vi "ReadText.vi"(8 "error in (no error)":errorcluster caption="错误输入（无错误）", 11 "zsActor输入":refnum<class "zsActor.lvclass">) -> (0 "error out":errorcluster caption="错误输出", 2 "Text":refnum<user-event>, 3 "zsActor输出":refnum<class "zsActor.lvclass">)   [LabVIEW 2014, in "Wrapper.lvlib" / "zsActor.lvclass"]
uses:
  zsActor.lvclass
  zsActor.lvclass/zsActor.ctl
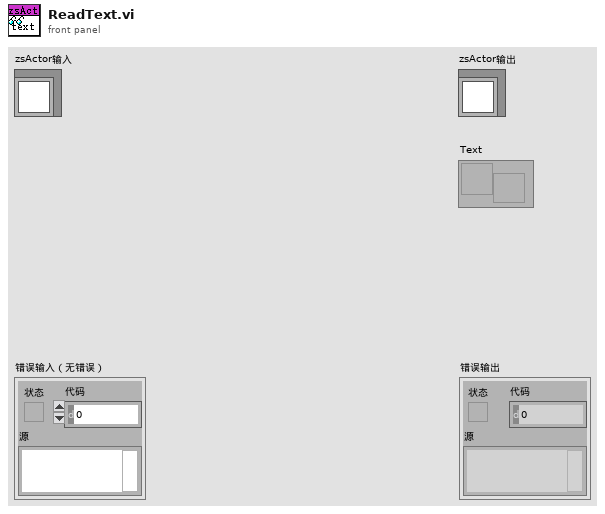
[diagram p1: front panel]
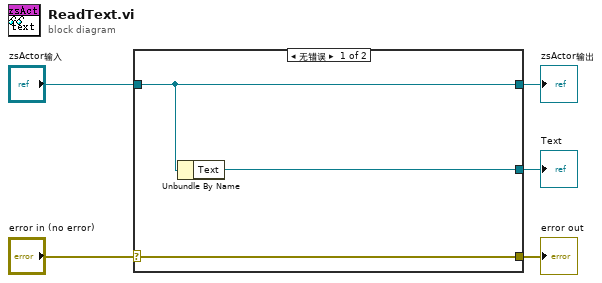
[diagram p0: block diagram]
diagram:
  n1 = case shown="无错误" "error in (no error)" {
    selector: "error in (no error)" -> [w8 w9]
    tunnel: [w8 w9] -> w4
    tunnel: [w7 w10] -> w2
    tunnel: "zsActor输入" -> [w7 w10]
    tunnel: [w6 _] -> w1
    frame No Error {
      n2 = Unbundle By Name(w7) -> ("Text"=w6:refnum<user-event>)
    }
    frame Error {
    }
  }
  "error out" <- w4
  "zsActor输出" <- w2
  "Text" <- w1
